vi "FP_Enable Disable Hide Control.vi"(6 "Settings":T2, 8 "Error":errorcluster, 11 "Ctl Refnum":refnum<vi>) -> (0 "Error Out":errorcluster, 1 "Disabled":T1(ring), 2 "Visible Out":bool, 3 "Ctl Refnum Out":refnum<vi>, 5 "Success":bool)   [LabVIEW 2020]
uses:
  TypeDefs_Utility/ENUM_FP_Hide Show Disable.ctl
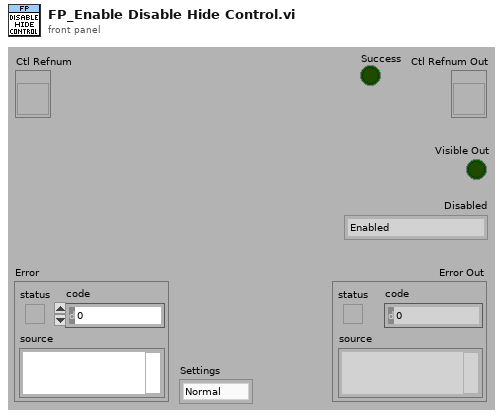
[diagram p1: front panel]
types:
  T1 = enum8{"Enabled", "Disabled", "Disabled and Grayed Out"}
  T2 = typedef "ENUM_FP_Hide Show Disable.ctl" = enum16{"Normal", "Disable", "Disable Gray", "Hide"}
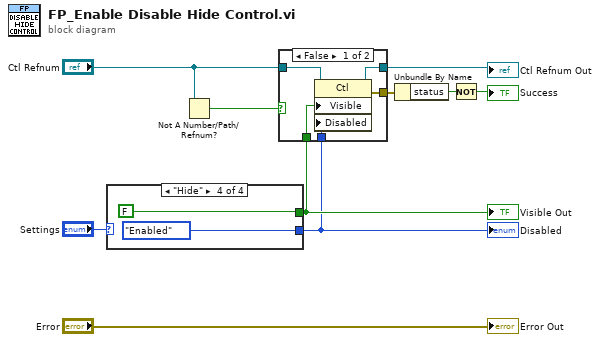
[diagram p0: block diagram]
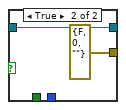
[diagram p2: hidden frame]
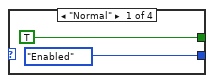
[diagram p3: hidden frame]
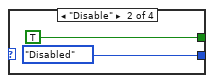
[diagram p4: hidden frame]
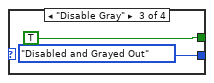
[diagram p5: hidden frame]
diagram:
  n1 = case shown="\"Hide\"" "Settings" {
    tunnel: [TRUE ("Visible") TRUE ("Visible") TRUE ("Visible") FALSE ("Visible")] -> w5
    tunnel: [T1."Enabled" ("Disabled") T1."Disabled" ("Disabled") T1."Disabled and Grayed Out" ("Disabled") T1."Enabled" ("Disabled")] -> w1
    frame "Normal" {
    }
    frame "Disable" {
    }
    frame "Disable Gray" {
    }
    frame "Hide" {
    }
  }
  "Visible Out" <- w5
  "Disabled" <- w1
  n2 = Not A Number/Path/Refnum?(number/path/refnum="Ctl Refnum") -> (NaN/Path/Refnum?=w8:bool)
  n3 = case shown="False" w8 {
    tunnel: "Ctl Refnum" -> [w23 w25]
    tunnel: [w22 w25] -> w6
    tunnel: w5 -> [w21 _]
    tunnel: w1 -> [w20 _]
    tunnel: [w19 errorcluster {"status"=FALSE, "code"=0, "source"=""} ("error out")] -> w3
    frame False {
      n4 = property class="Ctl"(reference=w23, "Visible"=w21, "Disabled"=w20) -> (reference out=w22:refnum<vi>, error out=w19:errorcluster)  [unwired: 1 in]
    }
    frame True {
    }
  }
  "Ctl Refnum Out" <- w6
  n5 = Unbundle By Name(w3) -> ("status"=w4:bool)
  n6 = Not(x=w4) -> (.not. x?=→"Success":bool)
  "Error Out" <- "Error"
